vi "Get Attribute as JSON.vi"(8 "error in":errorcluster, 10 "Attribute":string="$", 11 "Config from Excel Table in":refnum<class "Config from Excel Table.lvclass">) -> (0 "error out":errorcluster, 2 "<JSON>":string, 3 "Config from Excel Table out":refnum<class "Config from Excel Table.lvclass">)   [LabVIEW 2025, in "Config from Excel Table.lvclass"]
uses:
  Config from Excel Table.lvclass
  Config from Excel Table.lvclass/Config from Excel Table.ctl
  fa7c44a9-9914-4245-a91d-d6219db658f3.vi
  <vilib>/Utility/error.llb/Trim Whitespace One-Sided.vi
  <vilib>/JDP Science/JSONtext/Variant to JSON Text.vi
  <vilib>/JDP Science/JSONtext/support/Format JSON Array Text.vi
  <vilib>/JDP Science/JSONtext/support/Format JSON Object.vi
  <vilib>/JDP Science/JSONtext/LVClass Serializer/JSONtext LVClass Serializer.lvclass
  <vilib>/JDP Science/JSONtext/JSONtext.lvlib
  <vilib>/Peter/Open Xml/Source/Open Xml.lvlib
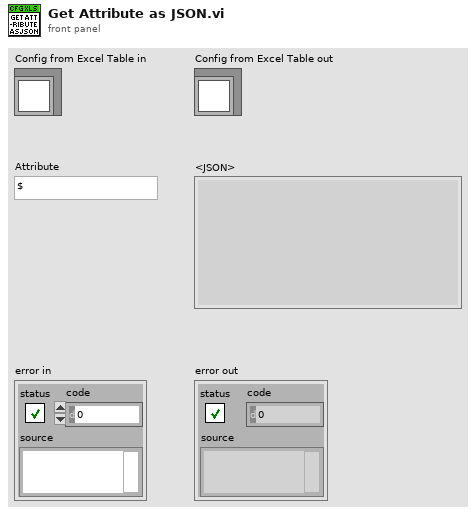
[diagram p1: front panel]
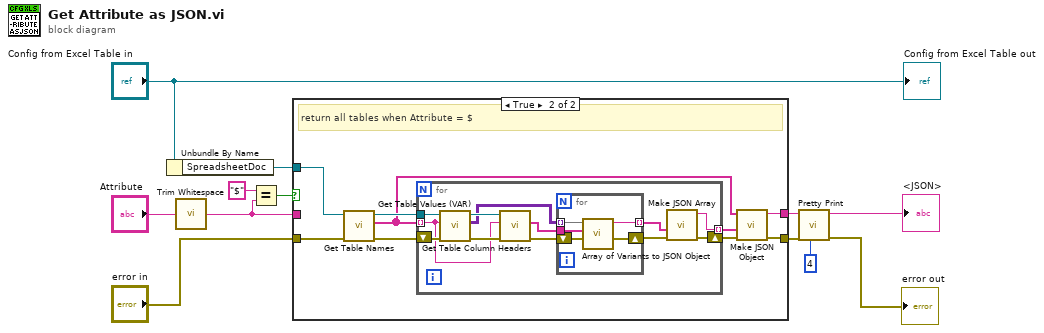
[diagram p0: block diagram]
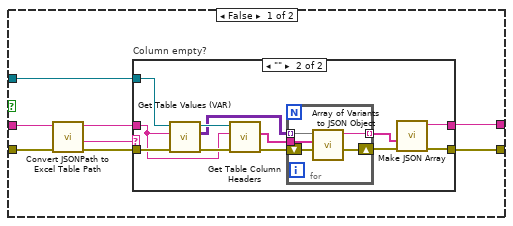
[diagram p2: hidden frame]
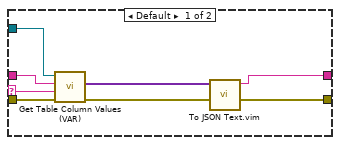
[diagram p3: hidden frame]
diagram:
  n1 = Unbundle By Name("Config from Excel Table in") -> ("SpreadsheetDoc"=w7:refnum<k24>)
  n2 = call <vilib>:"Trim Whitespace.vi"("string"="Attribute") -> ("trimmed string"=w1:string)  [unwired: 1 in]
  n3 = Equal?(x="$", y=w1) -> (x = y?=w4:bool)
  n4 = case shown="True" w4 {
    tunnel: w1 -> [w20 _]
    tunnel: "error in" -> [w19 w54]
    tunnel: w7 -> [w17 w53]
    tunnel: [w15 w49] -> w6
    tunnel: [w14 w46] -> w5
    frame False {
      n5 = call "Convert JSONPath to Excel Table Path.vi"("error in"=w19, "JSONPath"=w20) -> ("error out"=w18:errorcluster, "Column"=w13:string, "Table Name"=w16:string)  [unwired: 6 in, 1 out]
      n6 = case "Column empty?" shown="\"\"" w13 {
        selector: w13 -> [w23 _]
        tunnel: w18 -> [w28 w40]
        tunnel: [w22 w30] -> w15
        tunnel: w17 -> [w27 w39]
        tunnel: w16 -> [w26 w35]
        tunnel: [w21 w29] -> w14
        frame Default {
          n7 = call <vilib>:"Get Table Column Values (VAR).vi"("error in"=w28, "Column Name"=w23, "Table Name"=w26, "SpreadsheetDoc in"=w27) -> ("error out"=w24:errorcluster, "Column Values"=w25:variant[])  [unwired: 5 in, 1 out]
          n8 = call "To JSON Text.vim"("error in (no error)"=w24, "Anything"=w25) -> ("error out"=w22:errorcluster, "<JSON>"=w21:string)  [unwired: 8 in]
        }
        frame "" {
          n9 = call <vilib>:"Get Table Values (VAR).vi"("error in"=w40, "Table Name"=w35, "SpreadsheetDoc in"=w39) -> ("error out"=w38:errorcluster, "Table Values"=w33:variant[][], "SpreadsheetDoc out"=w36:refnum<k24>)  [unwired: 6 in]
          n10 = call <vilib>:"Get Table Column Headers.vi"("error in"=w38, "Table Name"=w35, "SpreadsheetDoc in"=w36) -> ("error out"=w37:errorcluster, "Headers"=w34:string[])  [unwired: 5 in, 2 out]
          n11 = for {
            tunnel: w34 -> [w44]
            tunnel: w33 -> [w43] mode=indexing
            shift-right: [w42] -> w31
            shift-left: w37 -> [w45]
            tunnel: [w41] -> w32 mode=indexing
            n12 = call <vilib>:"Array of Variants to JSON Object.vi"("error in (no error)"=w45, "Names"=w44, "Array"=w43) -> ("error out"=w42:errorcluster, "<JSON>"=w41:string)  [unwired: 7 in]
          }
          n13 = call <vilib>:"Make JSON Array.vi"("error in (no error)"=w31, "JSON Elements"=w32) -> ("error out"=w30:errorcluster, "<JSON>"=w29:string)  [unwired: 8 in]
        }
      }
    }
    frame True {
      # "return all tables when Attribute = $"
      n14 = call <vilib>:"Get Table Names.vi"("error in"=w54, "SpreadsheetDoc in"=w53) -> ("error out"=w52:errorcluster, "Table Names"=w47:string[], "SpreadsheetDoc out"=w51:refnum<k24>)  [unwired: 6 in, 1 out]
      n15 = for {
        tunnel: w47 -> [w55] mode=indexing
        tunnel: w51 -> [w57]
        tunnel: [w56] -> w48 mode=indexing
        shift-right: [w58] -> w50
        shift-left: w52 -> [w59]
        n16 = call <vilib>:"Get Table Values (VAR).vi"("error in"=w59, "Table Name"=w55, "SpreadsheetDoc in"=w57) -> ("error out"=w66:errorcluster, "Table Values"=w62:variant[][], "SpreadsheetDoc out"=w64:refnum<k24>)  [unwired: 6 in]
        n17 = call <vilib>:"Get Table Column Headers.vi"("error in"=w66, "Table Name"=w55, "SpreadsheetDoc in"=w64) -> ("error out"=w65:errorcluster, "Headers"=w63:string[])  [unwired: 5 in, 2 out]
        n18 = for {
          tunnel: w63 -> [w70]
          tunnel: w62 -> [w69] mode=indexing
          shift-right: [w68] -> w60
          shift-left: w65 -> [w71]
          tunnel: [w67] -> w61 mode=indexing
          n19 = call <vilib>:"Array of Variants to JSON Object.vi"("error in (no error)"=w71, "Names"=w70, "Array"=w69) -> ("error out"=w68:errorcluster, "<JSON>"=w67:string)  [unwired: 7 in]
        }
        n20 = call <vilib>:"Make JSON Array.vi"("error in (no error)"=w60, "JSON Elements"=w61) -> ("error out"=w58:errorcluster, "<JSON>"=w56:string)  [unwired: 8 in]
      }
      n21 = call <vilib>:"Make JSON Object.vi"("error in (no error)"=w50, "JSON Items"=w48, "Item Names"=w47) -> ("error out"=w49:errorcluster, "<JSON>"=w46:string)  [unwired: 7 in]
    }
  }
  n22 = call <vilib>:"Pretty Print.vi"("Pretty Print Levels"=4, "error in (no error)"=w6, "JSON"=w5) -> ("error out"=→"error out":errorcluster, "<JSON>"=→"<JSON>":string)  [unwired: 6 in, 1 out]
  "Config from Excel Table out" <- "Config from Excel Table in"
